vi "test Counter Pulse Width.vi"(8 "error in (no error)":errorcluster, 11 "TestCase in":refnum<class "Scan Engine cRIO System Tests.lvclass">) -> (0 "error out":errorcluster, 3 "TestCase out":refnum<class "Scan Engine cRIO System Tests.lvclass">)   [LabVIEW 2016, in "Scan Engine cRIO System Tests.lvclass"]
uses:
  Scan Engine cRIO System Tests.lvclass
  C:/Users/rzoeller/Documents/ni-official/niveristand-custom-device-testing-tools/VeriStandTestCase/VeriStandTestCase.lvclass
  <vilib>/addons/_JKI Toolkits/VI Tester/TestCase.llb/TestCase.lvclass
  niveristand-custom-device-testing-tools/VeriStandTestCase/VeriStandTestCase.lvclass
  C:/Program Files (x86)/National Instruments/LabVIEW 2016/vi.lib/addons/_JKI Toolkits/VI Tester/TestCase.llb/TestCase.lvclass
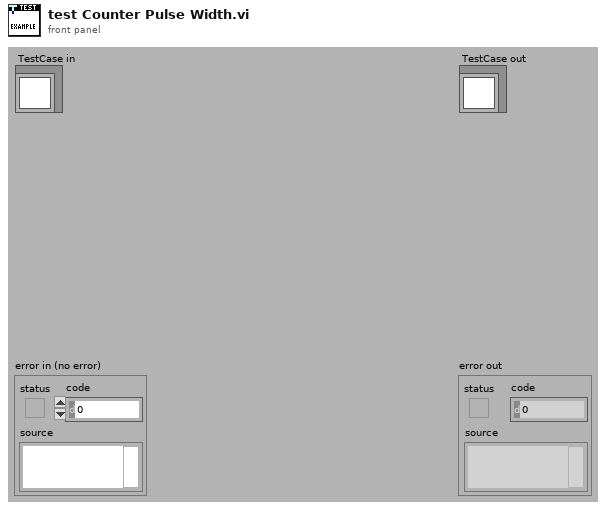
[diagram p1: front panel]
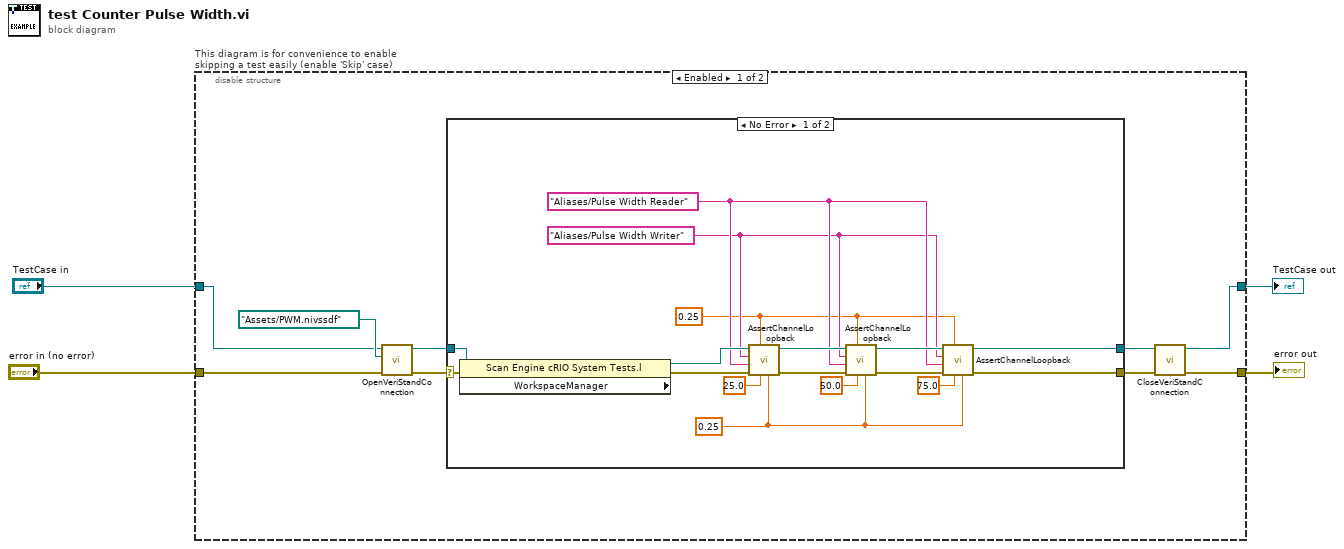
[diagram p0: block diagram]
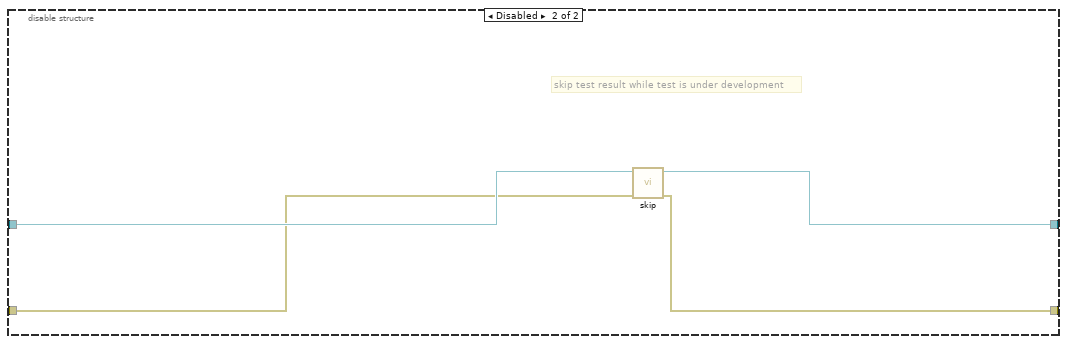
[diagram p3: hidden frame]
diagram:
  n1 = disable-structure "This diagram is for convenience to enable skipping a test easily (enable 'Skip' case)" shown="Enabled" {
    disable-tunnel: "TestCase in" -> [w9 w36]
    disable-tunnel: [w5 w34] -> w1
    disable-tunnel: [w7 w35] -> w3
    disable-tunnel: "error in (no error)" -> [w11 w33]
    frame Enabled {
      n2 = call-dynamic "OpenVeriStandConnection.vi"("error in (no error)"=w11, "System Definition File"=path "Assets/PWM.nivssdf", "VeriStand Test Case in"=w9) -> ("error out"=w12:errorcluster, "VeriStand Test Case out"=w10:refnum<class "Scan Engine cRIO System Tests.lvclass">)  [unwired: 7 in]
      n3 = case shown="No Error" w12 {
        selector: w12 -> [w30 w32]
        tunnel: [w19 w32] -> w8
        tunnel: [w21 w31] -> w6
        tunnel: w10 -> [w29 w31]
        frame No Error {
          w14 = 0.25 ("Delay Time (s)")
          w16 = 0.25 ("Tolerance")
          w17 = "Aliases/Pulse Width Writer" ("Channel")
          w18 = "Aliases/Pulse Width Reader" ("Channel")
          n4 = property class="Scan Engine cRIO System Tests.l" props=["WorkspaceManager"](reference=w29, error in=w30) -> (reference out=w28:refnum<class "Scan Engine cRIO System Tests.lvclass">, error out=w27:errorcluster)  [unwired: 1 out]
          n5 = call "AssertChannelLoopback.vi"("Tolerance"=w16, "Value"=25.0, "Delay Time (s)"=w14, "error in (no error)"=w27, "Read Channel"=w18, "Write Channel"=w17, "VeriStand Test Case in"=w28) -> ("error out"=w24:errorcluster, "VeriStand Test Case out"=w25:refnum<class "Scan Engine cRIO System Tests.lvclass">)  [unwired: 3 in]
          n6 = call "AssertChannelLoopback.vi"("Tolerance"=w16, "Value"=50.0, "Delay Time (s)"=w14, "error in (no error)"=w24, "Read Channel"=w18, "Write Channel"=w17, "VeriStand Test Case in"=w25) -> ("error out"=w20:errorcluster, "VeriStand Test Case out"=w22:refnum<class "Scan Engine cRIO System Tests.lvclass">)  [unwired: 3 in]
          n7 = call "AssertChannelLoopback.vi"("Tolerance"=w16, "Value"=75.0, "Delay Time (s)"=w14, "error in (no error)"=w20, "Read Channel"=w18, "Write Channel"=w17, "VeriStand Test Case in"=w22) -> ("error out"=w19:errorcluster, "VeriStand Test Case out"=w21:refnum<class "Scan Engine cRIO System Tests.lvclass">)  [unwired: 3 in]
        }
        frame Error {
        }
      }
      n8 = call-dynamic "CloseVeriStandConnection.vi"("error in (no error)"=w8, "VeriStand Test Case in"=w6) -> ("error out"=w7:errorcluster, "VeriStand Test Case out"=w5:refnum<class "Scan Engine cRIO System Tests.lvclass">)  [unwired: 8 in]
    }
    frame Disabled {
      # "skip test result while test is under development"
      n9 = call <vilib>:"skip.vi"("error in (no error)"=w33, "TestCase in"=w36) -> ("error out"=w35:errorcluster, "TestCase out"=w34:refnum<class "Scan Engine cRIO System Tests.lvclass">)  [unwired: 8 in]
    }
  }
  "error out" <- w3
  "TestCase out" <- w1
